vi "Get Score.vi"(11 "Submission in":refnum<class "Submission.lvclass">) -> (2 "Score":T1, 3 "Submission out":refnum<class "Submission.lvclass">)   [LabVIEW 2020, in "Summer of LabVIEW.lvlib" / "Submission.lvclass"]
uses:
  Submission.lvclass
  Submission.lvclass/Submission.ctl
  SoL Scoring/Score Entry.ctl
  SoL Scoring/SoL Scoring.lvlib
  SoL Scoring/Score.ctl
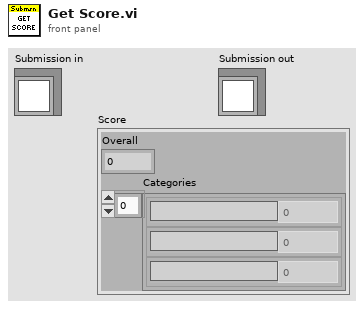
[diagram p1: front panel]
types:
  T1 = typedef "SoL Scoring.lvlib/Score.ctl" = cluster{"Overall":dbl, "Categories":T2[]}
  T2 = typedef "SoL Scoring.lvlib/Score Entry.ctl" = cluster{"Category":string, "Value":dbl}
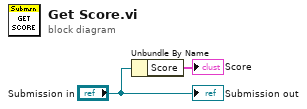
[diagram p0: block diagram]
diagram:
  n1 = Unbundle By Name("Submission in") -> ("Score"=→"Score":T1)
  "Submission out" <- "Submission in"
